vi "Convert to PWM Module.vi"(8 "error in":errorcluster, 9 "SD Module in":refnum<class "SD Module.lvclass">, 10 "slot ref in":T1 format="%.0x", 11 "module in":refnum<class "Module.lvclass">) -> (0 "error out":errorcluster, 1 "SD Module out":refnum<class "SD Module.lvclass">, 2 "slot ref out":T1 format="%.0x", 3 "module out":refnum<class "Module.lvclass">)   [LabVIEW 2017, in "Scan Engine Scripting.lvlib"]
uses:
  Scan Engine Scripting.lvlib
  Modules.lvlibp/SD Module/SD Module.lvclass
  Modules/Module/Module.lvclass
  <vilib>/NI Veristand/Custom Device API/Custom Device Item Ref.ctl
  Modules/Mode Classes/PWM Mode/PWM Mode.lvclass
  C:/dev/github.com/debryant/niveristand-scan-engine-ethercat-custom-device/Custom Device Source/Scripting/Modules/Mode Classes/Mode/Mode.lvclass
  476ebf56-c544-4016-8b90-3ae33c18c92c.vi
  Modules/Channel Classes/PWM Channel/PWM Channel.lvclass
  C:/dev/github.com/debryant/niveristand-scan-engine-ethercat-custom-device/Custom Device Source/Scripting/Modules/Channel Classes/Channel/Channel.lvclass
  Modules/Mode Classes/Create Mode.vi
  Modules/Mode Classes/PWM Mode/Create PWM Mode.vi
  <vilib>/NI Veristand/Custom Device API/Custom Device API.lvlib
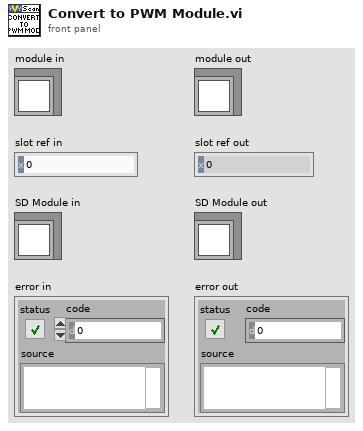
[diagram p1: front panel]
types:
  T1 = typedef "Custom Device API.lvlib/Custom Device Item Ref.ctl" = u64
  T2 = typedef "Scan Engine Scripting.lvlib/pwm channel settings.ctl" = cluster{"name":string, "default value":dbl, "frequency":T3}
  T3 = typedef "Scan Engine Scripting.lvlib/PWM Output Channel.lvclass/Frequency.ctl" = enum16{"1 Hz (1,000,000 us)", "50 Hz (20,000 us)", "250 Hz (4,000 us)", "500 Hz (2,000 us)", "1 kHz (1,000 us)", "5 kHz (200 us)", "10 kHz (100 us)", "20 kHz (50 us)"}
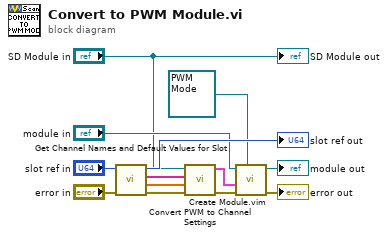
[diagram p0: block diagram]
diagram:
  n1 = call "Get Channel Names and Default Values for Slot.vi"("error in"="error in", "slot ref in"="slot ref in") -> ("error out"=w7:errorcluster, "channel default values"=w5:dbl[], "channel names"=w6:string[], "slot ref out"=→"slot ref out":T1)  [unwired: 6 in]
  n2 = call "Convert PWM to Channel Settings.vi"("error in"=w7, "channel default values"=w5, "channel names"=w6, "SD Module in"="SD Module in") -> ("error out"=w10:errorcluster, "channel settings"=w2:T2[])  [unwired: 6 in]
  n3 = call "Create Module.vim"("mode in"=refnum<class "PWM Mode.lvclass"> refnum ("Scan Engine Scripting.lvlib:PWM Mode.lvclass"), "error in"=w10, "channel settings"=w2, "module in"="module in") -> ("error out"=→"error out":errorcluster, "module out"=→"module out":refnum<class "Module.lvclass">)  [unwired: 6 in]
  "SD Module out" <- "SD Module in"
